vi "Configure Continuous Time Linear Equalizer.vi"(0 "VISA resource name":refnum<visa-resource-name>, 1 "Scale Mode (0: Auto)":i32(ring) items=["Auto", "Manual"], 2 "Enable CTLE (F: Disable)":bool, 5 "Source (0: Channel 1)":i32(ring) items=["Channel 1", "Channel 2", "Channel 3", "Channel 4", "Function 1", "Function 2", "Function 3", "Function 4", "Memory 1", "Memory 2", "Memory 3", "Memory 4"], 7 "DC Gain (0.667)":dbl=0.667, 9 "Data Rate (1E+9)":dbl=1000000000.0, 11 "error in (no error)":errorcluster, 12 "CTLE Vertical Offset (0 volt)":dbl, 13 "CTLE Vertical Range (64)":i32=64) -> (4 "VISA resource name out":refnum<visa-resource-name>, 15 "error out":errorcluster)   [LabVIEW 2020, in "Agilent 90000 Series.lvlib"]
doc: "Configures the basic settings for continuous time linear equalizer."
uses:
  Agilent 90000 Series.lvlib
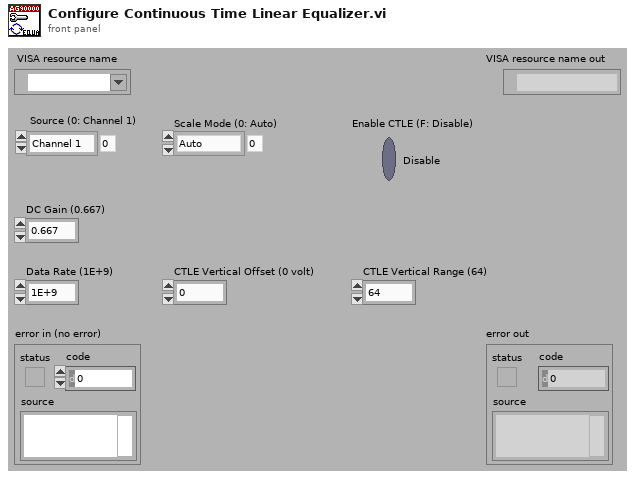
[diagram p1: front panel]
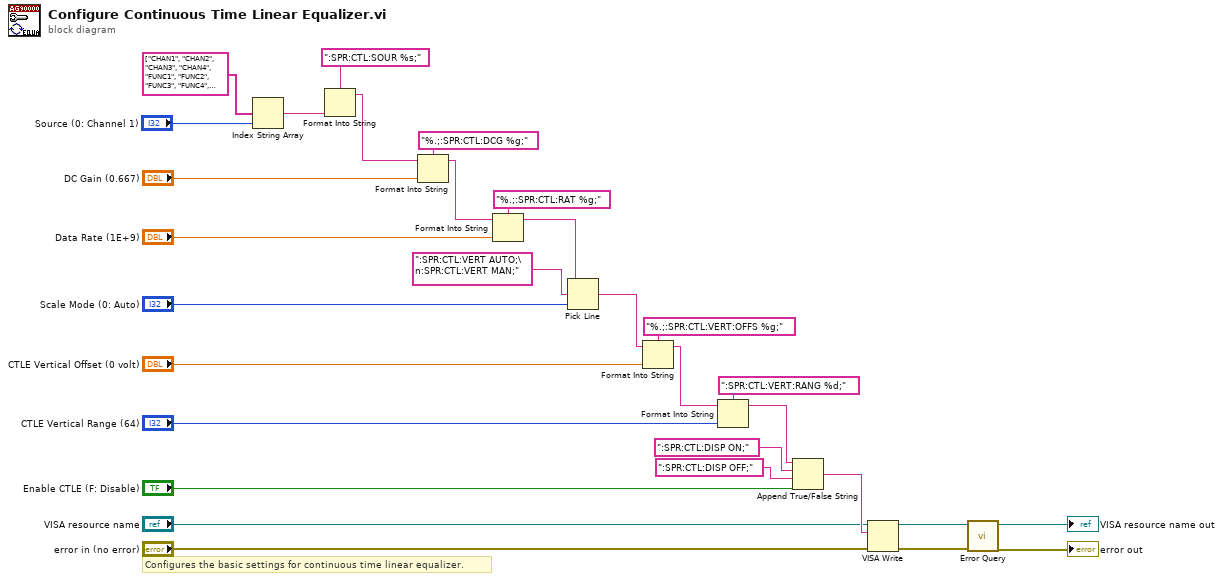
[diagram p0: block diagram]
diagram:
  # "Configures the basic settings for continuous time linear equalizer."
  n1 = Index String Array(1:"Source (0: Channel 1)", 2:string[] ["CHAN1", "CHAN2", "CHAN3", "CHAN4", "FUNC1", "FUNC2", "FUNC3", "FUNC4", "WMEM1", "WMEM2", "WMEM3", "WMEM4"]) -> (0:w2:string)  [unwired: 1 out]
  n2 = Format Into String(format string=":SPR:CTL:SOUR %s;", w2) -> (resulting string=w1:string)  [unwired: 2 in, 1 out]
  n3 = Format Into String(format string="%.;:SPR:CTL:DCG %g;", initial string=w1, "DC Gain (0.667)") -> (resulting string=w28:string)  [unwired: 1 in, 1 out]
  n4 = Format Into String(format string="%.;:SPR:CTL:RAT %g;", initial string=w28, "Data Rate (1E+9)") -> (resulting string=w23:string)  [unwired: 1 in, 1 out]
  n5 = Pick Line(string ("")=w23, multi-line string=":SPR:CTL:VERT AUTO;\n:SPR:CTL:VERT MAN;", line index="Scale Mode (0: Auto)") -> (output string=w22:string)
  n6 = Format Into String(format string="%.;:SPR:CTL:VERT:OFFS %g;", initial string=w22, "CTLE Vertical Offset (0 volt)") -> (resulting string=w19:string)  [unwired: 1 in, 1 out]
  n7 = Format Into String(format string=":SPR:CTL:VERT:RANG %d;", initial string=w19, "CTLE Vertical Range (64)") -> (resulting string=w16:string)  [unwired: 1 in, 1 out]
  n8 = Append True/False String(1:"Enable CTLE (F: Disable)", 2:":SPR:CTL:DISP OFF;", 3:":SPR:CTL:DISP ON;", 4:w16) -> (0:w12:string)
  n9 = VISA Write(VISA resource name="VISA resource name", write buffer=w12, error in (no error)="error in (no error)") -> (VISA resource name out=w9:refnum<visa-resource-name>, error out=w8:errorcluster)  [unwired: 1 out]
  n10 = call "Error Query.vi"("error in (no error)"=w8, "VISA resource name"=w9) -> ("error out"=→"error out":errorcluster, "VISA resource name out"=→"VISA resource name out":refnum<visa-resource-name>)  [unwired: 8 out]
